vi "XLP80_EA_Run Devices.vi"(8 "err in":errorcluster, 10 "Device Informations":T1, 11 "Simu EAs":T2) -> (0 "Error EAs":T3, 2 "Device Informations OUT":T1)   [LabVIEW 2021]
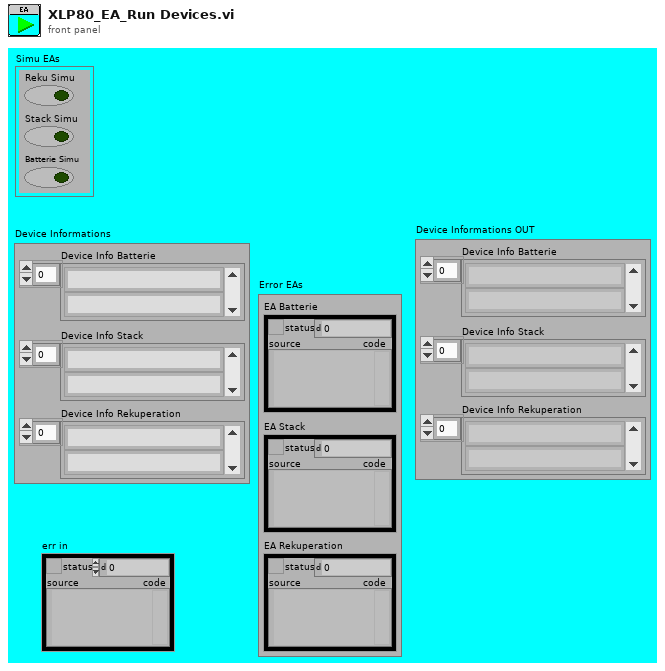
[diagram p1: front panel]
types:
  T1 = cluster{"Device Info Batterie":string[], "Device Info Stack":string[], "Device Info Rekuperation":string[]}
  T2 = cluster{"Reku Simu":bool, "Stack Simu":bool, "Batterie Simu":bool}
  T3 = cluster{"EA Batterie":errorcluster, "EA Stack":errorcluster, "EA Rekuperation":errorcluster}
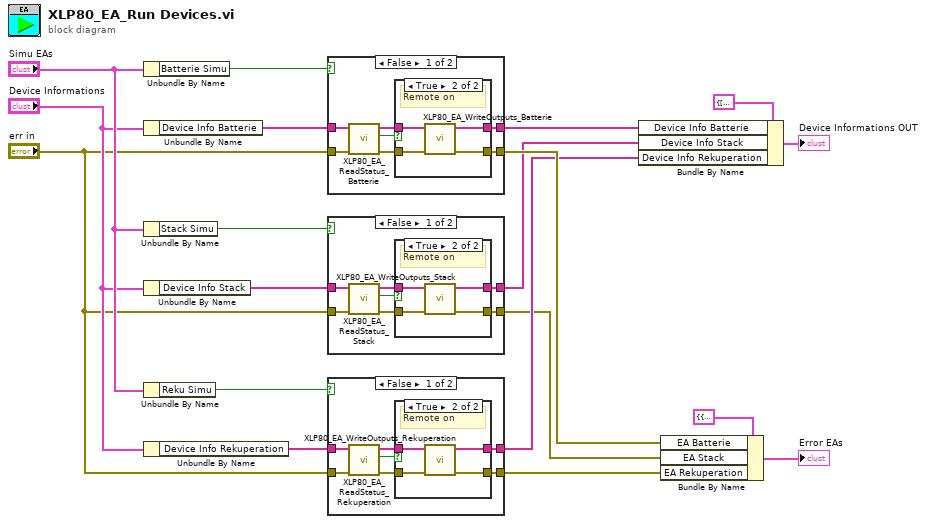
[diagram p0: block diagram]
diagram:
  n1 = Unbundle By Name("Simu EAs") -> ("Batterie Simu"=w15:bool)
  n2 = Unbundle By Name("Device Informations") -> ("Device Info Batterie"=w14:string[])
  n3 = Unbundle By Name("Simu EAs") -> ("Stack Simu"=w9:bool)
  n4 = Unbundle By Name("Device Informations") -> ("Device Info Stack"=w8:string[])
  n5 = Unbundle By Name("Simu EAs") -> ("Reku Simu"=w6:bool)
  n6 = Unbundle By Name("Device Informations") -> ("Device Info Rekuperation"=w5:string[])
  n7 = case shown="False" w15 {
    tunnel: [w26 w33] -> w13
    tunnel: [w25 w34] -> w10
    tunnel: "err in" -> [w24 w33]
    tunnel: w14 -> [w21 w34]
    frame False {
      n8 = call "XLP80_EA_ReadStatus_Batterie.vi"("err in"=w24, "Device information"=w21) -> ("err out"=w23:errorcluster, "Remote ON"=w22:bool, "Device information IN"=w20:string[])  [unwired: 7 in]
      n9 = case shown="True" w22 {
        tunnel: w20 -> [w28 w32]
        tunnel: w23 -> [w27 w31]
        tunnel: [w27 w30] -> w26
        tunnel: [w28 w29] -> w25
        frame False {
          # "remote Off"
        }
        frame True {
          # "Remote on"
          n10 = call "XLP80_EA_WriteOutputs_Batterie.vi"("err in"=w31, "Device information"=w32) -> ("err out"=w30:errorcluster, "Device information IN"=w29:string[])  [unwired: 8 in]
        }
      }
    }
    frame True {
    }
  }
  n11 = case shown="False" w9 {
    tunnel: [w41 w48] -> w2
    tunnel: [w40 w49] -> w7
    tunnel: "err in" -> [w39 w48]
    tunnel: w8 -> [w36 w49]
    frame False {
      n12 = call "XLP80_EA_ReadStatus_Stack.vi"("err in"=w39, "Device information"=w36) -> ("err out"=w38:errorcluster, "Remote ON"=w37:bool, "Device information IN"=w35:string[])  [unwired: 7 in]
      n13 = case shown="True" w37 {
        tunnel: w35 -> [w43 w47]
        tunnel: w38 -> [w42 w46]
        tunnel: [w42 w45] -> w41
        tunnel: [w43 w44] -> w40
        frame False {
          # "remote Off"
        }
        frame True {
          # "Remote on"
          n14 = call "XLP80_EA_WriteOutputs_Stack.vi"("err in"=w46, "Device information"=w47) -> ("err out"=w45:errorcluster, "Device information IN"=w44:string[])  [unwired: 8 in]
        }
      }
    }
    frame True {
    }
  }
  n15 = case shown="False" w6 {
    tunnel: [w56 w63] -> w1
    tunnel: [w55 w64] -> w3
    tunnel: "err in" -> [w54 w63]
    tunnel: w5 -> [w51 w64]
    frame False {
      n16 = call "XLP80_EA_ReadStatus_Rekuperation.vi"("err in"=w54, "Device information"=w51) -> ("err out"=w53:errorcluster, "Remote ON"=w52:bool, "Device information IN"=w50:string[])  [unwired: 7 in]
      n17 = case shown="True" w52 {
        tunnel: w50 -> [w58 w62]
        tunnel: w53 -> [w57 w61]
        tunnel: [w57 w60] -> w56
        tunnel: [w58 w59] -> w55
        frame False {
          # "remote Off"
        }
        frame True {
          # "Remote on"
          n18 = call "XLP80_EA_WriteOutputs_Rekuperation.vi"("err in"=w61, "Device information"=w62) -> ("err out"=w60:errorcluster, "Device information IN"=w59:string[])  [unwired: 8 in]
        }
      }
    }
    frame True {
    }
  }
  n19 = Bundle By Name(cluster=T1 {"Device Info Batterie"=[], "Device Info Stack"=[], "Device Info Rekuperation"=[]} ("Device Informations"), "Device Info Batterie"=w10, "Device Info Stack"=w7, "Device Info Rekuperation"=w3) -> (→"Device Informations OUT":T1)
  n20 = Bundle By Name(cluster=T3 {"EA Batterie"={"status"=FALSE, "code"=0, "source"=""}, "EA Stack"={"status"=FALSE, "code"=0, "source"=""}, "EA Rekuperation"={"status"=FALSE, "code"=0, "source"=""}} ("Error EAs"), "EA Batterie"=w13, "EA Stack"=w2, "EA Rekuperation"=w1) -> (→"Error EAs":T3)
